vi "Write Handle.vi"(8 "error in (no error)":errorcluster, 11 "Channel in":refnum<class "Channel.lvclass">) -> (0 "error out":errorcluster, 3 "Channel out":refnum<class "Channel.lvclass">)   [LabVIEW 2018, in "Channel.lvclass"]
uses:
  Channel.lvclass
  Channel.lvclass/Channel.ctl
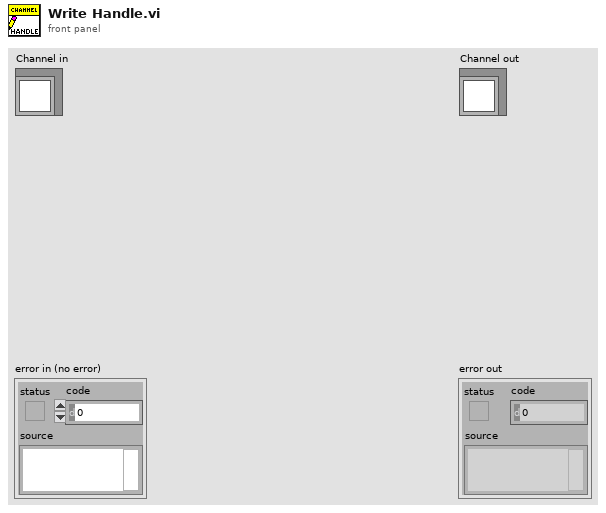
[diagram p1: front panel]
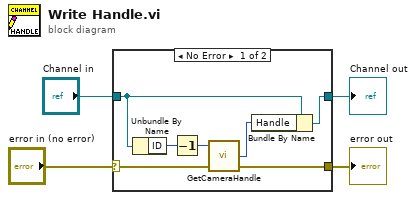
[diagram p0: block diagram]
diagram:
  n1 = case shown="No Error" "error in (no error)" {
    selector: "error in (no error)" -> [w10 w12]
    tunnel: [w9 w12] -> w3
    tunnel: [w11 w13] -> w1
    tunnel: "Channel in" -> [w7 w13]
    frame No Error {
      n2 = Unbundle By Name(w7) -> ("ID"=w6:u8)
      n3 = Decrement(x=w6) -> (x-1=w5:u8)
      n4 = call <userlib>:"GetCameraHandle.vi"("error in (no error)"=w10, "cameraIndex"=w5) -> ("error out"=w9:errorcluster, "cameraHandle"=w8:i32)  [unwired: 1 in, 1 out]
      n5 = Bundle By Name(cluster=w7, "Handle"=w8) -> (w11:refnum<class "Channel.lvclass">)
    }
    frame Error {
    }
  }
  "error out" <- w3
  "Channel out" <- w1
